vi "Source Controller.vi"() -> ()   [LabVIEW 2015]
uses:
  Type/_PIC Channel.ctl
  Type/_RT Command.ctl
  <vilib>/Utility/config.llb/Read Key (Boolean).vi
  <vilib>/Utility/config.llb/Read Key (I32).vi
  <vilib>/Utility/config.llb/Write Key (Boolean).vi
  <vilib>/Utility/config.llb/Write Key (U32).vi
  <vilib>/Utility/config.llb/NI_LVConfig.lvlib
panel:
  out "Src 2 -HV Mon":u16
  in  "Source 2 -HV":u16
  out "Src 1 -HV Mon":u16
  in  "Source 1 -HV":u16
  out "Curtain-HV Mon":u16
  in  "Curtain Cap -HV":u16
  out "Corona-HV Mon":u16
  in  "Corona -HV":u16
  out "Test":bool
  out "quit":bool
  in  "Test Channel":T1(ring)
  out "Current Cycle #":i32
  in  "# of Cycles":i32=100
  in  "Ramp Down T (mS)":u32=100
  in  "Ramp Up T (mS)":u32=100
  in  "Start Test":bool
  in  "CEM Pol":bool
  out "String":string
  in  "Pol Switch":bool
  in  "Current Channel":T2
  out "I/O Port Hd 4":u16 format="%.0x"
  out "I/O Port 4 Mon":u16
  in  "Time Const 4":u16
  out "I/O Port Hd 3":u16 format="%.0x"
  out "I/O Port 3 Mon":u16
  in  "Time Const 3":u16
  out "I/O Port Hd 2":u16 format="%.0x"
  out "I/O Port 2 Mon":u16
  in  "Time Const 2":u16
  out "I/O Port Hd 1":u16 format="%.0x"
  out "I/O Port 1 Mon":u16
  in  "Time Const 1":u16
  out "Source 2 Temp Hd":u16 format="%.0x"
  out "Source 2 HV Hd":u16 format="%.0x"
  out "Source 1 Temp Hd":u16 format="%.0x"
  out "Source 1 HV Hd":u16 format="%.0x"
  out "Curtain Cap HV Hd":u16 format="%.0x"
  out "HSID Temp Hd":u16 format="%.0x"
  out "Corona HV Hd":u16 format="%.0x"
  out "Src 2 Temp Mon":u16
  in  "Source 2 Temp":u16
  out "Src 2 +HV Mon":u16
  in  "Source 2 +HV":u16
  out "Src 1 Temp Mon":u16
  in  "Source 1 Temp":u16
  out "Src 1 +HV Mon":u16
  in  "Source 2 Pol":bool
  in  "Source 1 Pol":bool
  in  "Update All":bool
  in  "Source 1 +HV":u16
  out "Curtain+HV Mon":u16
  in  "Curtain Cap +HV":u16
  out "HSID Temp Mon":u16
  in  "HSID Temp":u16
  out "Corona+HV Mon":u16
  in  "Curtain Cap Pol":bool
  in  "Corona Pol":bool
  in  "EL":bool=TRUE
  in  "Update 1":bool
  in  "Corona +HV":u16
  in  "RP":bool=TRUE
  in  "Abort Test":bool
  # "HSID"
  # "Dual Source"
  # "HV Switch Test"
  # "Choose a Test Channel and enter the test voltages in the appropriate boxes above then press Start Test"
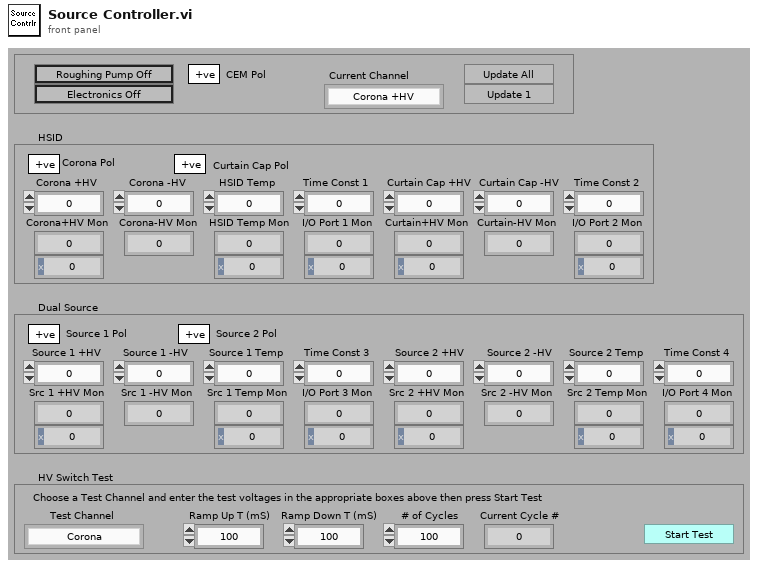
[diagram p1: front panel]
types:
  T1 = enum16{"Corona", "Curtain Cap", "Source 1", "Source 2"}
  T2 = typedef "_PIC Channel.ctl" = enum16{"Corona +HV", "Corona -HV", "HSID Temp", "Time Const 1", "Curtain Cap +HV", "Curtain Cap -HV", "Time Const 2", "Source 1 +HV", "Source 1 -HV", "Source 1 Temp", "Time Const 3", "Source 2 +HV", "Source 2 -HV", "Source 2 Temp", "Time Const 4"}
  T3 = typedef "_RT Command.ctl" = enum16{"xml Start Run", "xml Start Actual Run", "xml Stop Run", "xml Runtime Update", "xml Get Status", "xml Get Table", "xml Set Table", "xml Get Configuration", "xml System Status", "xml Set LC Input Logic", "xml Get Data", "xml Get Info", "Start", "StartActualRun", "Stop", "Runtime Update", "Get Data", "Get Info", "Get Status", "Get Param", "Get Config", "Get Table", "Read ADC", "Set Oscillator", "Update Config", "Update Table", "Set All Pol", "Set Pol and DC", "Set Max Mass", "Toggle RP", "Toggle EL", "Set PIC", "Initialize Turbo", "Send Turbo Comm", "Close Turbo", "P1", "P2", "P3", "Send Serial", "Set LC Out", "Get LC In", "Read VAC", "Test Table", "Toggle Power", "Get Startup", "Set Startup", "Get ADC Table", "Set ADC Table", "Get Brief Status", "Get Detail Status", "Auxiliary Update", "Set CC Logics", "Set CC Input Logics", "Ignore Error", "invalid"}
  T4 = typedef "NI_LVConfig.lvlib/Config Data RefNum.ctl" = refnum<k1>
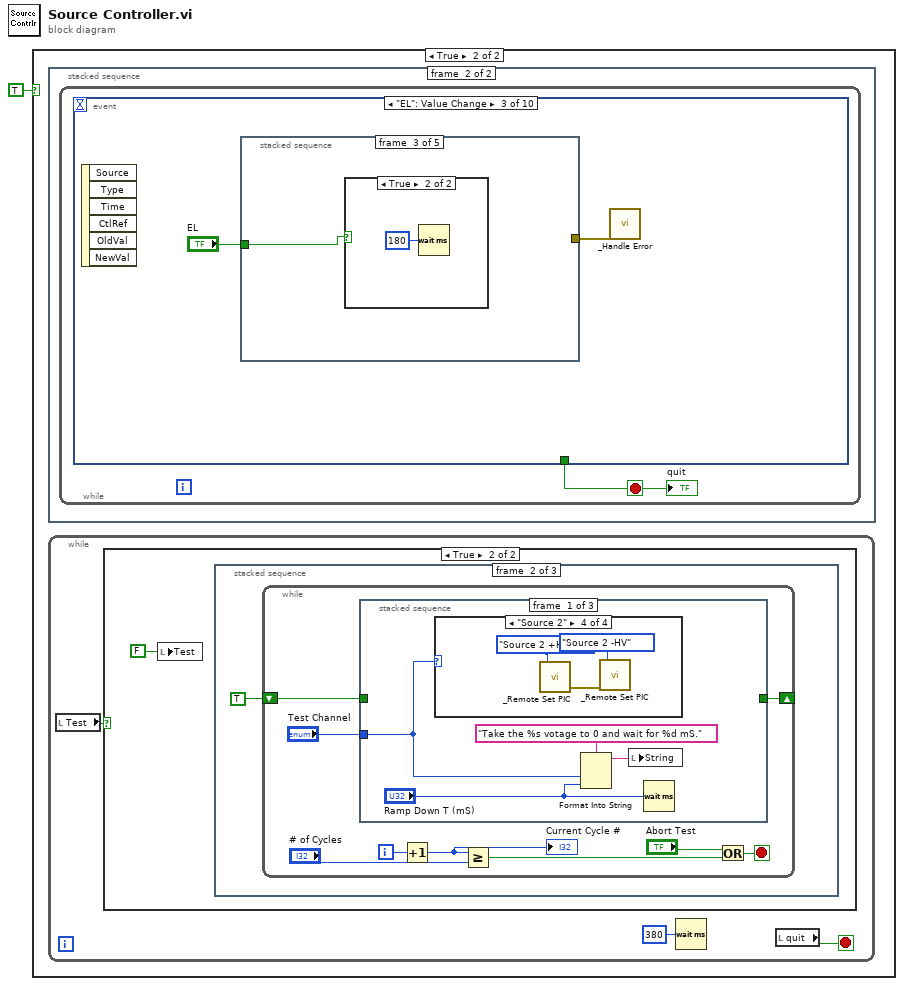
[diagram p0: block diagram]
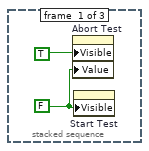
[diagram p4: hidden frame]
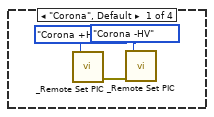
[diagram p5: hidden frame]
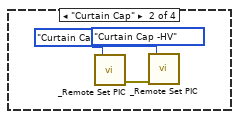
[diagram p6: hidden frame]
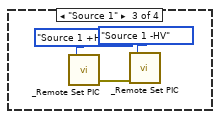
[diagram p7: hidden frame]
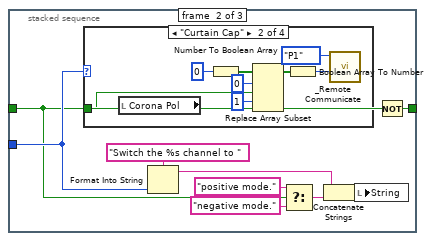
[diagram p8: hidden frame]
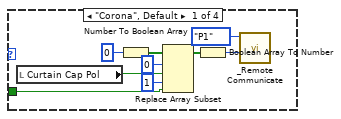
[diagram p9: hidden frame]
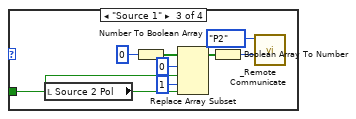
[diagram p10: hidden frame]
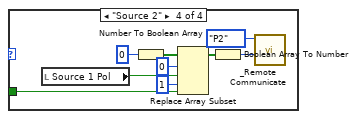
[diagram p11: hidden frame]
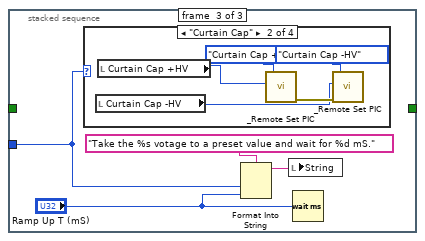
[diagram p12: hidden frame]
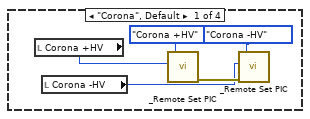
[diagram p13: hidden frame]
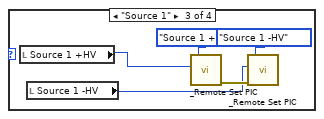
[diagram p14: hidden frame]
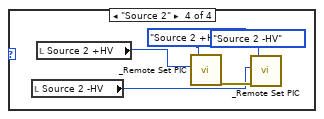
[diagram p15: hidden frame]
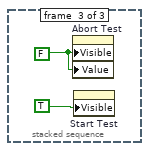
[diagram p16: hidden frame]
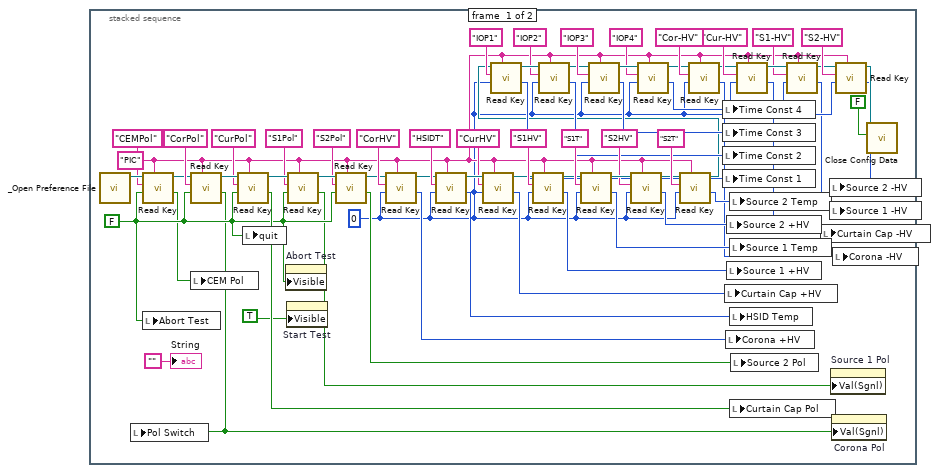
[diagram p17: hidden frame]
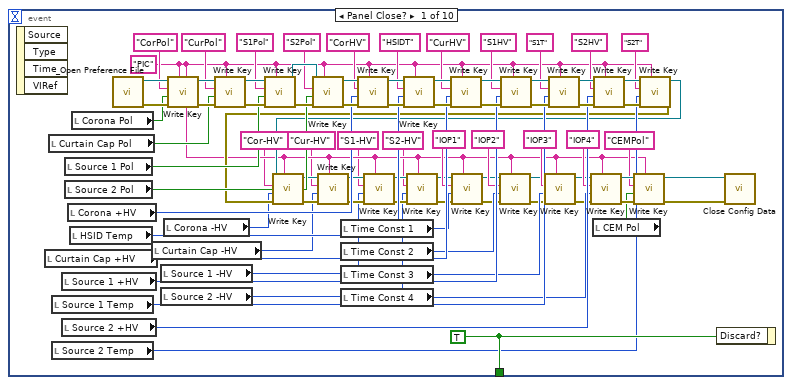
[diagram p18: hidden frame]
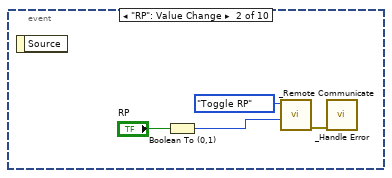
[diagram p19: hidden frame]
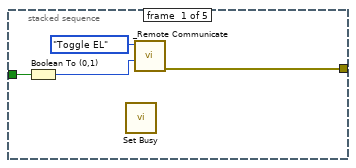
[diagram p20: hidden frame]
diagram:
  n1 = case shown="True" TRUE {
    frame False {
    }
    frame True {
      n2 = stacked-sequence {
        frame #0 {
          w123 = FALSE
          w112 = 0
          w114 = "PIC" ("section")
          n3 = call "_Open Preference File.vi"() -> ("refnum"=w128:T4)  [unwired: 3 in, 4 out]
          n4 = call-poly <vilib>:"Read Key.vi"("section"=w114, "default value"=w123, "key"="CEMPol" ("section"), "refnum"=w128) -> ("value"=w107:bool, "refnum out"=w127:T4)  [unwired: 1 in, 5 out]
          n5 = local write "Abort Test"(w123) -> ()
          n6 = call-poly <vilib>:"Read Key.vi"("section"=w114, "default value"=w123, "key"="CorPol" ("section"), "refnum"=w127) -> ("value"=w106:bool, "refnum out"=w170:T4)  [unwired: 1 in, 5 out]
          n7 = local write "Pol Switch"(w106) -> ()
          n8 = local write "CEM Pol"(w107) -> ()
          n9 = call-poly <vilib>:"Read Key.vi"("section"=w114, "default value"=w123, "key"="CurPol" ("section"), "refnum"=w170) -> ("value"=w142:bool, "refnum out"=w169:T4)  [unwired: 1 in, 5 out]
          n10 = local write "quit"(w123) -> ()
          n11 = property on="Abort Test" class="Bool (strict)"("Visible"=w123) -> ()  [unwired: 2 in, 2 out]
          n12 = property on="Start Test" class="Bool"("Visible"=TRUE) -> ()  [unwired: 2 in, 2 out]
          n13 = call-poly <vilib>:"Read Key.vi"("section"=w114, "default value"=w123, "key"="S1Pol" ("section"), "refnum"=w169) -> ("value"=w105:bool, "refnum out"=w168:T4)  [unwired: 1 in, 5 out]
          n14 = call-poly <vilib>:"Read Key.vi"("section"=w114, "default value"=w123, "key"="S2Pol" ("section"), "refnum"=w168) -> ("value"=w143:bool, "refnum out"=w162:T4)  [unwired: 1 in, 5 out]
          n15 = call-poly <vilib>:"Read Key.vi"("section"=w114, "default value"=w112, "key"="CorHV" ("section"), "refnum"=w162) -> ("value"=w144:i32, "refnum out"=w153:T4)  [unwired: 1 in, 5 out]
          n16 = call-poly <vilib>:"Read Key.vi"("section"=w114, "default value"=w112, "key"="HSIDT" ("section"), "refnum"=w153) -> ("value"=w145:i32, "refnum out"=w155:T4)  [unwired: 1 in, 5 out]
          n17 = call-poly <vilib>:"Read Key.vi"("section"=w114, "default value"=w112, "key"="CurHV" ("section"), "refnum"=w155) -> ("value"=w146:i32, "refnum out"=w156:T4)  [unwired: 1 in, 5 out]
          n18 = call-poly <vilib>:"Read Key.vi"("section"=w114, "default value"=w112, "key"="S1HV" ("section"), "refnum"=w156) -> ("value"=w147:i32, "refnum out"=w157:T4)  [unwired: 1 in, 5 out]
          n19 = call-poly <vilib>:"Read Key.vi"("section"=w114, "default value"=w112, "key"="S1T" ("section"), "refnum"=w157) -> ("value"=w148:i32, "refnum out"=w161:T4)  [unwired: 1 in, 5 out]
          n20 = call-poly <vilib>:"Read Key.vi"("section"=w114, "default value"=w112, "key"="S2HV" ("section"), "refnum"=w161) -> ("value"=w149:i32, "refnum out"=w151:T4)  [unwired: 1 in, 5 out]
          n21 = call-poly <vilib>:"Read Key.vi"("section"=w114, "default value"=w112, "key"="S2T" ("section"), "refnum"=w151) -> ("value"=w150:i32, "refnum out"=w130:T4)  [unwired: 1 in, 5 out]
          n22 = call-poly <vilib>:"Read Key.vi"("section"=w114, "default value"=w112, "key"="IOP1" ("section"), "refnum"=w130) -> ("value"=w131:i32, "refnum out"=w139:T4)  [unwired: 1 in, 5 out]
          n23 = call-poly <vilib>:"Read Key.vi"("section"=w114, "default value"=w112, "key"="IOP2" ("section"), "refnum"=w139) -> ("value"=w132:i32, "refnum out"=w135:T4)  [unwired: 1 in, 5 out]
          n24 = call-poly <vilib>:"Read Key.vi"("section"=w114, "default value"=w112, "key"="IOP3" ("section"), "refnum"=w135) -> ("value"=w133:i32, "refnum out"=w141:T4)  [unwired: 1 in, 5 out]
          n25 = call-poly <vilib>:"Read Key.vi"("section"=w114, "default value"=w112, "key"="IOP4" ("section"), "refnum"=w141) -> ("value"=w125:i32, "refnum out"=w115:T4)  [unwired: 1 in, 5 out]
          n26 = call-poly <vilib>:"Read Key.vi"("section"=w114, "default value"=w112, "key"="Cor-HV" ("section"), "refnum"=w115) -> ("value"=w108:i32, "refnum out"=w118:T4)  [unwired: 1 in, 5 out]
          n27 = local write "Time Const 4"(w125) -> ()
          n28 = local write "Time Const 3"(w133) -> ()
          n29 = local write "Time Const 2"(w132) -> ()
          n30 = local write "Time Const 1"(w131) -> ()
          n31 = local write "Curtain Cap +HV"(w146) -> ()
          n32 = local write "Corona +HV"(w144) -> ()
          n33 = local write "Source 2 +HV"(w149) -> ()
          n34 = local write "Source 1 +HV"(w147) -> ()
          n35 = local write "Source 2 Temp"(w150) -> ()
          n36 = local write "Source 1 Temp"(w148) -> ()
          n37 = local write "HSID Temp"(w145) -> ()
          n38 = local write "Curtain Cap Pol"(w142) -> ()
          n39 = local write "Source 2 Pol"(w143) -> ()
          n40 = call-poly <vilib>:"Read Key.vi"("section"=w114, "default value"=w112, "key"="Cur-HV" ("section"), "refnum"=w118) -> ("value"=w109:i32, "refnum out"=w122:T4)  [unwired: 1 in, 5 out]
          n41 = call-poly <vilib>:"Read Key.vi"("section"=w114, "default value"=w112, "key"="S1-HV" ("section"), "refnum"=w122) -> ("value"=w110:i32, "refnum out"=w116:T4)  [unwired: 1 in, 5 out]
          n42 = local write "Curtain Cap -HV"(w109) -> ()
          n43 = local write "Source 1 -HV"(w110) -> ()
          n44 = property on="Source 1 Pol" class="Bool (strict)"("Val(Sgnl)"=w105) -> ()  [unwired: 2 in, 2 out]
          n45 = property on="Corona Pol" class="Bool (strict)"("Val(Sgnl)"=w106) -> ()  [unwired: 2 in, 2 out]
          n46 = local write "Corona -HV"(w108) -> ()
          n47 = call-poly <vilib>:"Read Key.vi"("section"=w114, "default value"=w112, "key"="S2-HV" ("section"), "refnum"=w116) -> ("value"=w111:i32, "refnum out"=w113:T4)  [unwired: 1 in, 5 out]
          n48 = local write "Source 2 -HV"(w111) -> ()
          n49 = call <vilib>:"Close Config Data.vi"("write file if changed (T)"=FALSE ("write configuration file? (T)"), "refnum"=w113) -> ()  [unwired: 1 in, 9 out]
          "String" <- ""
        }
        frame #1 {
          n50 = while {
            stop <- w172 stop-if-true
            n51 = event shown="[2] \"EL\": Value Change" {
              selector: _ -> [_ _ _ _ _ _ _ _ _ _]
              dyn-events: _ -> [_ _ _ _ _ _ _ _ _ _]
              timeout: _ -> [_ _ _ _ _ _ _ _ _ _]
              tunnel: [w256 _ _ _ _ _ _ _ _ _] -> w172
              event Panel Close? {
                w181 = "PIC" ("section")
                w256 = TRUE
                n52 = event-data() -> ()  [unwired: 5 out]
                n53 = local read "Curtain Cap +HV"() -> (w216:u16)
                n54 = local read "Curtain Cap Pol"() -> (w221:bool)
                n55 = local read "Source 1 Temp"() -> (w214:u16)
                n56 = local read "Source 2 Temp"() -> (w212:u16)
                n57 = local read "Source 1 +HV"() -> (w215:u16)
                n58 = local read "Source 2 +HV"() -> (w213:u16)
                n59 = local read "Source 1 Pol"() -> (w220:bool)
                n60 = local read "Source 2 Pol"() -> (w219:bool)
                n61 = local read "Corona +HV"() -> (w218:u16)
                n62 = local read "HSID Temp"() -> (w217:u16)
                n63 = local read "Corona Pol"() -> (w222:bool)
                n64 = call "_Open Preference File.vi"() -> ("error"=w252:errorcluster, "refnum"=w251:T4)  [unwired: 3 in, 3 out]
                n65 = local read "Curtain Cap -HV"() -> (w175:u16)
                n66 = local read "Source 1 -HV"() -> (w174:u16)
                n67 = local read "Source 2 -HV"() -> (w173:u16)
                n68 = local read "Corona -HV"() -> (w176:u16)
                n69 = call-poly <vilib>:"Write Key.vi"("section"=w181, "error in (no error)"=w252, "value"=w222, "key"="CorPol" ("section"), "refnum"=w251) -> ("error out"=w253:errorcluster, "refnum out"=w250:T4)  [unwired: 5 out]
                n70 = call-poly <vilib>:"Write Key.vi"("section"=w181, "error in (no error)"=w253, "value"=w221, "key"="CurPol" ("section"), "refnum"=w250) -> ("error out"=w254:errorcluster, "refnum out"=w249:T4)  [unwired: 5 out]
                n71 = call-poly <vilib>:"Write Key.vi"("section"=w181, "error in (no error)"=w254, "value"=w220, "key"="S1Pol" ("section"), "refnum"=w249) -> ("error out"=w255:errorcluster, "refnum out"=w248:T4)  [unwired: 5 out]
                n72 = call-poly <vilib>:"Write Key.vi"("section"=w181, "error in (no error)"=w255, "value"=w219, "key"="S2Pol" ("section"), "refnum"=w248) -> ("error out"=w246:errorcluster, "refnum out"=w247:T4)  [unwired: 5 out]
                n73 = local read "Time Const 1"() -> (w204:u16)
                n74 = local read "Time Const 2"() -> (w203:u16)
                n75 = local read "Time Const 3"() -> (w202:u16)
                n76 = local read "Time Const 4"() -> (w201:u16)
                n77 = call-poly <vilib>:"Write Key.vi"("section"=w181, "error in (no error)"=w246, "value"=w218, "key"="CorHV" ("section"), "refnum"=w247) -> ("error out"=w237:errorcluster, "refnum out"=w236:T4)  [unwired: 5 out]
                n78 = call-poly <vilib>:"Write Key.vi"("section"=w181, "error in (no error)"=w237, "value"=w217, "key"="HSIDT" ("section"), "refnum"=w236) -> ("error out"=w240:errorcluster, "refnum out"=w241:T4)  [unwired: 5 out]
                n79 = call-poly <vilib>:"Write Key.vi"("section"=w181, "error in (no error)"=w240, "value"=w216, "key"="CurHV" ("section"), "refnum"=w241) -> ("error out"=w239:errorcluster, "refnum out"=w242:T4)  [unwired: 5 out]
                n80 = call-poly <vilib>:"Write Key.vi"("section"=w181, "error in (no error)"=w239, "value"=w215, "key"="S1HV" ("section"), "refnum"=w242) -> ("error out"=w238:errorcluster, "refnum out"=w243:T4)  [unwired: 5 out]
                n81 = call-poly <vilib>:"Write Key.vi"("section"=w181, "error in (no error)"=w238, "value"=w214, "key"="S1T" ("section"), "refnum"=w243) -> ("error out"=w245:errorcluster, "refnum out"=w244:T4)  [unwired: 5 out]
                n82 = local read "CEM Pol"() -> (w194:bool)
                n83 = call-poly <vilib>:"Write Key.vi"("section"=w181, "error in (no error)"=w245, "value"=w213, "key"="S2HV" ("section"), "refnum"=w244) -> ("error out"=w235:errorcluster, "refnum out"=w234:T4)  [unwired: 5 out]
                n84 = call-poly <vilib>:"Write Key.vi"("section"=w181, "error in (no error)"=w235, "value"=w212, "key"="S2T" ("section"), "refnum"=w234) -> ("error out"=w184:errorcluster, "refnum out"=w183:T4)  [unwired: 5 out]
                n85 = call-poly <vilib>:"Write Key.vi"("section"=w181, "error in (no error)"=w184, "value"=w176, "key"="Cor-HV" ("section"), "refnum"=w183) -> ("error out"=w191:errorcluster, "refnum out"=w190:T4)  [unwired: 5 out]
                n86 = call-poly <vilib>:"Write Key.vi"("section"=w181, "error in (no error)"=w191, "value"=w175, "key"="Cur-HV" ("section"), "refnum"=w190) -> ("error out"=w186:errorcluster, "refnum out"=w187:T4)  [unwired: 5 out]
                n87 = call-poly <vilib>:"Write Key.vi"("section"=w181, "error in (no error)"=w186, "value"=w174, "key"="S1-HV" ("section"), "refnum"=w187) -> ("error out"=w189:errorcluster, "refnum out"=w188:T4)  [unwired: 5 out]
                n88 = call-poly <vilib>:"Write Key.vi"("section"=w181, "error in (no error)"=w189, "value"=w173, "key"="S2-HV" ("section"), "refnum"=w188) -> ("error out"=w185:errorcluster, "refnum out"=w182:T4)  [unwired: 5 out]
                n89 = call-poly <vilib>:"Write Key.vi"("section"=w181, "error in (no error)"=w185, "value"=w204, "key"="IOP1" ("section"), "refnum"=w182) -> ("error out"=w200:errorcluster, "refnum out"=w206:T4)  [unwired: 5 out]
                n90 = call-poly <vilib>:"Write Key.vi"("section"=w181, "error in (no error)"=w200, "value"=w203, "key"="IOP2" ("section"), "refnum"=w206) -> ("error out"=w199:errorcluster, "refnum out"=w205:T4)  [unwired: 5 out]
                n91 = call-poly <vilib>:"Write Key.vi"("section"=w181, "error in (no error)"=w199, "value"=w202, "key"="IOP3" ("section"), "refnum"=w205) -> ("error out"=w198:errorcluster, "refnum out"=w207:T4)  [unwired: 5 out]
                n92 = call-poly <vilib>:"Write Key.vi"("section"=w181, "error in (no error)"=w198, "value"=w201, "key"="IOP4" ("section"), "refnum"=w207) -> ("error out"=w196:errorcluster, "refnum out"=w197:T4)  [unwired: 5 out]
                n93 = call-poly <vilib>:"Write Key.vi"("section"=w181, "error in (no error)"=w196, "value"=w194, "key"="CEMPol" ("section"), "refnum"=w197) -> ("error out"=w192:errorcluster, "refnum out"=w193:T4)  [unwired: 5 out]
                n94 = event-data("Discard?"=w256) -> ()  [unwired: 1 in, 1 out]
                n95 = call <vilib>:"Close Config Data.vi"("error in (no error)"=w192, "refnum"=w193) -> ()  [unwired: 1 in, 9 out]
              }
              event "RP": Value Change {
                n96 = event-data() -> ()  [unwired: 2 out]
                n97 = Boolean To (0,1)(Boolean="RP") -> (0, 1=w257:i16)
                n98 = call "_Remote Communicate.vi"("DC Param"=w257, "Command"=_RT_Command."Toggle RP") -> ("error out"=w259:errorcluster)  [unwired: 4 in, 3 out]
                n99 = call "_Handle Error.vi"("error in (no error)"=w259) -> ()  [unwired: 2 in, 5 out]
              }
              event "EL": Value Change {
                n100 = event-data() -> ()  [unwired: 7 out]
                n101 = stacked-sequence {
                  tunnel: "EL" -> [w265 w267 w270 w272 _]
                  tunnel: [w263 _ _ _ _] -> w261
                  frame #0 {
                    n102 = Boolean To (0,1)(Boolean=w265) -> (0, 1=w264:i16)
                    n103 = call <vilib>:"Set Busy.vi"() -> ()  [unwired: 4 in, 8 out]
                    n104 = call "_Remote Communicate.vi"("DC Param"=w264, "Command"=_RT_Command."Toggle EL") -> ("error out"=w263:errorcluster)  [unwired: 4 in, 3 out]
                  }
                  frame #1 {
                    n105 = case shown="True" w267 {
                      frame False {
                      }
                      frame True {
                        n106 = call "_Remote Park Lens.vi"("All Ch (F)"=TRUE) -> ("error out"=w268:errorcluster)  [unwired: 1 in, 5 out]
                        n107 = call "_Remote Program Oscil.vi"("error in (no error)"=w268) -> ()  [unwired: 1 out]
                      }
                    }
                  }
                  frame #2 {
                    n108 = case shown="True" w270 {
                      frame False {
                      }
                      frame True {
                        n109 = Wait (ms)(milliseconds to wait=u32 180) -> ()  [unwired: 1 out]
                      }
                    }
                  }
                  frame #3 {
                    n110 = case shown="True" w272 {
                      frame False {
                      }
                      frame True {
                        n111 = call "_Remote Park Lens.vi"("All Ch (F)"=TRUE) -> ("error out"=w273:errorcluster)  [unwired: 1 in, 5 out]
                        n112 = call "_Remote Program Oscil.vi"("error in (no error)"=w273) -> ()  [unwired: 1 out]
                      }
                    }
                  }
                  frame #4 {
                    n113 = call <vilib>:"Unset Busy.vi"() -> ()  [unwired: 2 in, 10 out]
                  }
                }
                n114 = call "_Handle Error.vi"("error in (no error)"=w261) -> ()  [unwired: 2 in, 5 out]
              }
              event "Update 1": Value Change {
                n115 = event-data() -> ()  [unwired: 7 out]
                n116 = stacked-sequence {
                  tunnel: [_ w280 _] -> w275
                  frame #0 {
                    n117 = call <vilib>:"Set Busy.vi"() -> ()  [unwired: 4 in, 8 out]
                  }
                  frame #1 {
                    n118 = case shown="\"Corona +HV\", Default" "Current Channel" {
                      tunnel: [w311 w312 w313 w314 w315 w316 w317 w318 w319 w320 w321 w322 w323 w324 w325] -> w276
                      frame "Corona +HV", Default {
                        n119 = local read "Corona +HV"() -> (w311:u16)
                      }
                      frame "Corona -HV" {
                        n120 = local read "Corona -HV"() -> (w312:u16)
                      }
                      frame "HSID Temp" {
                        n121 = local read "HSID Temp"() -> (w313:u16)
                      }
                      frame "Time Const 1" {
                        n122 = local read "Time Const 1"() -> (w314:u16)
                      }
                      frame "Curtain Cap +HV" {
                        n123 = local read "Curtain Cap +HV"() -> (w315:u16)
                      }
                      frame "Curtain Cap -HV" {
                        n124 = local read "Curtain Cap -HV"() -> (w316:u16)
                      }
                      frame "Time Const 2" {
                        n125 = local read "Time Const 2"() -> (w317:u16)
                      }
                      frame "Source 1 +HV" {
                        n126 = local read "Source 1 +HV"() -> (w318:u16)
                      }
                      frame "Source 1 -HV" {
                        n127 = local read "Source 1 -HV"() -> (w319:u16)
                      }
                      frame "Source 1 Temp" {
                        n128 = local read "Source 1 Temp"() -> (w320:u16)
                      }
                      frame "Time Const 3" {
                        n129 = local read "Time Const 3"() -> (w321:u16)
                      }
                      frame "Source 2 +HV" {
                        n130 = local read "Source 2 +HV"() -> (w322:u16)
                      }
                      frame "Source 2 -HV" {
                        n131 = local read "Source 2 -HV"() -> (w323:u16)
                      }
                      frame "Source 2 Temp" {
                        n132 = local read "Source 2 Temp"() -> (w324:u16)
                      }
                      frame "Time Const 4" {
                        n133 = local read "Time Const 4"() -> (w325:u16)
                      }
                    }
                    n134 = call "_Remote Set PIC.vi"("Set Value"=w276, "PIC Channel"="Current Channel") -> ("error out"=w280:errorcluster, "Received Value"=w277:u16, "Received Header"=w278:u16)  [unwired: 1 in, 2 out]
                    n135 = case shown="\"Source 2 Temp\"" "Current Channel" {
                      tunnel: w278 -> [w282 w284 w286 w288 w290 w292 w294 w296 w298 w300 w302 w304 w306 w308 w310]
                      tunnel: w277 -> [w281 w283 w285 w287 w289 w291 w293 w295 w297 w299 w301 w303 w305 w307 w309]
                      frame "Corona +HV", Default {
                        n136 = local write "Corona HV Hd"(w282) -> ()
                        n137 = local write "Corona+HV Mon"(w281) -> ()
                      }
                      frame "Corona -HV" {
                        n138 = local write "Corona HV Hd"(w284) -> ()
                        n139 = local write "Corona-HV Mon"(w283) -> ()
                      }
                      frame "HSID Temp" {
                        n140 = local write "HSID Temp Mon"(w285) -> ()
                        n141 = local write "HSID Temp Hd"(w286) -> ()
                      }
                      frame "Time Const 1" {
                        n142 = local write "I/O Port 1 Mon"(w287) -> ()
                        n143 = local write "I/O Port Hd 1"(w288) -> ()
                      }
                      frame "Curtain Cap +HV" {
                        n144 = local write "Curtain Cap HV Hd"(w290) -> ()
                        n145 = local write "Curtain+HV Mon"(w289) -> ()
                      }
                      frame "Curtain Cap -HV" {
                        n146 = local write "Curtain Cap HV Hd"(w292) -> ()
                        n147 = local write "Curtain-HV Mon"(w291) -> ()
                      }
                      frame "Time Const 2" {
                        n148 = local write "I/O Port 2 Mon"(w293) -> ()
                        n149 = local write "I/O Port Hd 2"(w294) -> ()
                      }
                      frame "Source 1 +HV" {
                        n150 = local write "Source 1 HV Hd"(w296) -> ()
                        n151 = local write "Src 1 +HV Mon"(w295) -> ()
                      }
                      frame "Source 1 -HV" {
                        n152 = local write "Source 1 HV Hd"(w298) -> ()
                        n153 = local write "Src 1 -HV Mon"(w297) -> ()
                      }
                      frame "Source 1 Temp" {
                        n154 = local write "Source 1 Temp Hd"(w300) -> ()
                        n155 = local write "Src 1 Temp Mon"(w299) -> ()
                      }
                      frame "Time Const 3" {
                        n156 = local write "I/O Port 3 Mon"(w301) -> ()
                        n157 = local write "I/O Port Hd 3"(w302) -> ()
                      }
                      frame "Source 2 +HV" {
                        n158 = local write "Source 2 HV Hd"(w304) -> ()
                        n159 = local write "Src 2 +HV Mon"(w303) -> ()
                      }
                      frame "Source 2 -HV" {
                        n160 = local write "Source 2 HV Hd"(w306) -> ()
                        n161 = local write "Src 2 -HV Mon"(w305) -> ()
                      }
                      frame "Source 2 Temp" {
                        n162 = local write "Source 2 Temp Hd"(w308) -> ()
                        n163 = local write "Src 2 Temp Mon"(w307) -> ()
                      }
                      frame "Time Const 4" {
                        n164 = local write "I/O Port 4 Mon"(w309) -> ()
                        n165 = local write "I/O Port Hd 4"(w310) -> ()
                      }
                    }
                  }
                  frame #2 {
                    n166 = call <vilib>:"Unset Busy.vi"() -> ()  [unwired: 2 in, 10 out]
                  }
                }
                n167 = call "_Handle Error.vi"("error in (no error)"=w275) -> ()  [unwired: 2 in, 5 out]
              }
              event "Update All": Value Change {
                n168 = event-data() -> ()  [unwired: 7 out]
                n169 = stacked-sequence {
                  frame #0 {
                    n170 = call <vilib>:"Set Busy.vi"() -> ()  [unwired: 4 in, 8 out]
                  }
                  frame #1 {
                    n171 = call "_Remote Set PIC.vi"("Set Value"="Corona +HV", "PIC Channel"=_PIC_Channel."Corona +HV") -> ("Received Value"=→"Corona+HV Mon":u16, "Received Header"=→"Corona HV Hd":u16)  [unwired: 1 in, 3 out]
                  }
                  frame #2 {
                    n172 = call "_Remote Set PIC.vi"("Set Value"="Corona -HV", "PIC Channel"=_PIC_Channel."Corona -HV") -> ("Received Value"=→"Corona-HV Mon":u16, "Received Header"=w330:u16)  [unwired: 1 in, 3 out]
                    n173 = local write "Corona HV Hd"(w330) -> ()
                  }
                  frame #3 {
                    n174 = call "_Remote Set PIC.vi"("Set Value"="HSID Temp", "PIC Channel"=_PIC_Channel."HSID Temp") -> ("Received Value"=→"HSID Temp Mon":u16, "Received Header"=→"HSID Temp Hd":u16)  [unwired: 1 in, 3 out]
                  }
                  frame #4 {
                    n175 = call "_Remote Set PIC.vi"("Set Value"="Time Const 1", "PIC Channel"=_PIC_Channel."Time Const 1") -> ("Received Value"=→"I/O Port 1 Mon":u16, "Received Header"=→"I/O Port Hd 1":u16)  [unwired: 1 in, 3 out]
                  }
                  frame #5 {
                    n176 = call "_Remote Set PIC.vi"("Set Value"="Curtain Cap +HV", "PIC Channel"=_PIC_Channel."Curtain Cap +HV") -> ("Received Value"=→"Curtain+HV Mon":u16, "Received Header"=→"Curtain Cap HV Hd":u16)  [unwired: 1 in, 3 out]
                  }
                  frame #6 {
                    n177 = call "_Remote Set PIC.vi"("Set Value"="Curtain Cap -HV", "PIC Channel"=_PIC_Channel."Curtain Cap -HV") -> ("Received Value"=→"Curtain-HV Mon":u16, "Received Header"=w347:u16)  [unwired: 1 in, 3 out]
                    n178 = local write "Curtain Cap HV Hd"(w347) -> ()
                  }
                  frame #7 {
                    n179 = call "_Remote Set PIC.vi"("Set Value"="Time Const 2", "PIC Channel"=_PIC_Channel."Time Const 2") -> ("Received Value"=→"I/O Port 2 Mon":u16, "Received Header"=→"I/O Port Hd 2":u16)  [unwired: 1 in, 3 out]
                  }
                  frame #8 {
                    n180 = call "_Remote Set PIC.vi"("Set Value"="Source 1 +HV", "PIC Channel"=_PIC_Channel."Source 1 +HV") -> ("Received Value"=→"Src 1 +HV Mon":u16, "Received Header"=→"Source 1 HV Hd":u16)  [unwired: 1 in, 3 out]
                  }
                  frame #9 {
                    n181 = call "_Remote Set PIC.vi"("Set Value"="Source 1 -HV", "PIC Channel"=_PIC_Channel."Source 1 -HV") -> ("Received Value"=→"Src 1 -HV Mon":u16, "Received Header"=w359:u16)  [unwired: 1 in, 3 out]
                    n182 = local write "Source 1 HV Hd"(w359) -> ()
                  }
                  frame #10 {
                    n183 = call "_Remote Set PIC.vi"("Set Value"="Source 1 Temp", "PIC Channel"=_PIC_Channel."Source 1 Temp") -> ("Received Value"=→"Src 1 Temp Mon":u16, "Received Header"=→"Source 1 Temp Hd":u16)  [unwired: 1 in, 3 out]
                  }
                  frame #11 {
                    n184 = call "_Remote Set PIC.vi"("Set Value"="Time Const 3", "PIC Channel"=_PIC_Channel."Time Const 3") -> ("Received Value"=→"I/O Port 3 Mon":u16, "Received Header"=→"I/O Port Hd 3":u16)  [unwired: 1 in, 3 out]
                  }
                  frame #12 {
                    n185 = call "_Remote Set PIC.vi"("Set Value"="Source 2 +HV", "PIC Channel"=_PIC_Channel."Source 2 +HV") -> ("Received Value"=→"Src 2 +HV Mon":u16, "Received Header"=→"Source 2 HV Hd":u16)  [unwired: 1 in, 3 out]
                  }
                  frame #13 {
                    n186 = call "_Remote Set PIC.vi"("Set Value"="Source 2 -HV", "PIC Channel"=_PIC_Channel."Source 2 -HV") -> ("Received Value"=→"Src 2 -HV Mon":u16, "Received Header"=w375:u16)  [unwired: 1 in, 3 out]
                    n187 = local write "Source 1 HV Hd"(w375) -> ()
                  }
                  frame #14 {
                    n188 = call "_Remote Set PIC.vi"("Set Value"="Source 2 Temp", "PIC Channel"=_PIC_Channel."Source 2 Temp") -> ("Received Value"=→"Src 2 Temp Mon":u16, "Received Header"=→"Source 2 Temp Hd":u16)  [unwired: 1 in, 3 out]
                  }
                  frame #15 {
                    n189 = call "_Remote Set PIC.vi"("Set Value"="Time Const 4", "PIC Channel"=_PIC_Channel."Time Const 4") -> ("Received Value"=→"I/O Port 4 Mon":u16, "Received Header"=→"I/O Port Hd 4":u16)  [unwired: 1 in, 3 out]
                  }
                  frame #16 {
                    n190 = call <vilib>:"Unset Busy.vi"() -> ()  [unwired: 2 in, 10 out]
                  }
                }
              }
              event "Pol Switch": Value Change {
                # "Obsolete"
                n191 = event-data() -> ()  [unwired: 7 out]
                n192 = stacked-sequence {
                  tunnel: "Pol Switch" -> [w387 _ _ w401 _ _]
                  frame #0 {
                    n193 = call <vilib>:"Set Busy.vi"() -> ()  [unwired: 4 in, 8 out]
                    n194 = local write "Curtain Cap Pol"(w387) -> ()
                    n195 = local write "Source 1 Pol"(w387) -> ()
                    n196 = local write "Corona Pol"(w387) -> ()
                    n197 = local write "Source 2 Pol"(w387) -> ()
                    n198 = local write "String"("Setting voltage to 0" ("String")) -> ()
                  }
                  frame #1 {
                    w389 = u16 0 ("Set Value")
                    n199 = call "_Remote Set PIC.vi"("Set Value"=w389, "PIC Channel"=_PIC_Channel."Corona +HV") -> ("error out"=w392:errorcluster)  [unwired: 1 in, 4 out]
                    n200 = call "_Remote Set PIC.vi"("error in (no error)"=w392, "Set Value"=w389, "PIC Channel"=_PIC_Channel."HSID Temp") -> ("error out"=w393:errorcluster)  [unwired: 4 out]
                    n201 = call "_Remote Set PIC.vi"("error in (no error)"=w393, "Set Value"=w389, "PIC Channel"=_PIC_Channel."Curtain Cap -HV") -> ("error out"=w394:errorcluster)  [unwired: 4 out]
                    n202 = call "_Remote Set PIC.vi"("error in (no error)"=w394, "Set Value"=w389, "PIC Channel"=_PIC_Channel."Source 1 -HV") -> ()  [unwired: 5 out]
                  }
                  frame #2 {
                    n203 = Wait (ms)(milliseconds to wait=u32 20000) -> ()  [unwired: 1 out]
                    n204 = local write "String"("Wait for 20 Sec" ("String")) -> ()
                  }
                  frame #3 {
                    n205 = Boolean To (0,1)(Boolean=w401) -> (0, 1=w400:i16)
                    n206 = local write "String"("Switching polarity" ("String")) -> ()
                    n207 = call "_Remote Communicate.vi"("DC Param"=w400, "Command"=_RT_Command."Set All Pol") -> ()  [unwired: 4 in, 4 out]
                  }
                  frame #4 {
                    n208 = local read "Curtain Cap +HV"() -> (w405:u16)
                    n209 = local read "Source 1 +HV"() -> (w404:u16)
                    n210 = local read "Source 2 +HV"() -> (w403:u16)
                    n211 = local read "Corona +HV"() -> (w406:u16)
                    n212 = call "_Remote Set PIC.vi"("Set Value"=w406, "PIC Channel"=_PIC_Channel."Corona +HV") -> ("error out"=w409:errorcluster)  [unwired: 1 in, 4 out]
                    n213 = call "_Remote Set PIC.vi"("error in (no error)"=w409, "Set Value"=w405, "PIC Channel"=_PIC_Channel."HSID Temp") -> ("error out"=w410:errorcluster)  [unwired: 4 out]
                    n214 = call "_Remote Set PIC.vi"("error in (no error)"=w410, "Set Value"=w404, "PIC Channel"=_PIC_Channel."Curtain Cap -HV") -> ("error out"=w411:errorcluster)  [unwired: 4 out]
                    n215 = call "_Remote Set PIC.vi"("error in (no error)"=w411, "Set Value"=w403, "PIC Channel"=_PIC_Channel."Source 1 -HV") -> ()  [unwired: 5 out]
                  }
                  frame #5 {
                    n216 = local write "String"("") -> ()
                    n217 = call <vilib>:"Unset Busy.vi"() -> ()  [unwired: 2 in, 10 out]
                  }
                }
              }
              event "Corona Pol", "Curtain Cap Pol": Value Change {
                n218 = event-data() -> ()  [unwired: 7 out]
                n219 = Number To Boolean Array(number=u16 0) -> (Boolean array=w422:bool[])
                n220 = Replace Array Subset(array=w422, new element #1="Curtain Cap Pol", index #1=0 ("index"), new element #2="Corona Pol", index #2=1 ("index")) -> (w419:bool[])
                n221 = Boolean Array To Number(Boolean array=w419) -> (number=w417:u16)
                n222 = call "_Remote Communicate.vi"("DC Param"=w417, "Command"=_RT_Command."P1") -> ()  [unwired: 4 in, 4 out]
              }
              event "Source 1 Pol", "Source 2 Pol": Value Change {
                n223 = event-data() -> ()  [unwired: 7 out]
                n224 = Number To Boolean Array(number=u16 0) -> (Boolean array=w431:bool[])
                n225 = Replace Array Subset(array=w431, new element #1="Source 1 Pol", index #1=0 ("index"), new element #2="Source 2 Pol", index #2=1 ("index")) -> (w428:bool[])
                n226 = Boolean Array To Number(Boolean array=w428) -> (number=w426:u16)
                n227 = call "_Remote Communicate.vi"("DC Param"=w426, "Command"=_RT_Command."P2") -> ()  [unwired: 4 in, 4 out]
              }
              event "CEM Pol": Value Change {
                n228 = event-data() -> ()  [unwired: 7 out]
                n229 = Number To Boolean Array(number=u16 0) -> (Boolean array=w439:bool[])
                n230 = Replace Array Subset(array=w439, new element #1="CEM Pol", index #1=0 ("index"), new element #2="CEM Pol", index #2=1 ("index")) -> (w436:bool[])
                n231 = Boolean Array To Number(Boolean array=w436) -> (number=w434:u16)
                n232 = call "_Remote Communicate.vi"("DC Param"=w434, "Command"=_RT_Command."P3") -> ()  [unwired: 4 in, 4 out]
              }
              event "Start Test": Value Change {
                n233 = event-data() -> ()  [unwired: 2 out]
                "Test" <- "Start Test"
              }
            }
            "quit" <- w172
          }
        }
      }
      n234 = while {
        stop <- w4 stop-if-true
        n235 = local read "Test"() -> (w2:bool)
        n236 = case shown="True" w2 {
          frame False {
          }
          frame True {
            n237 = local write "Test"(FALSE ("Test")) -> ()
            n238 = stacked-sequence {
              frame #0 {
                w6 = FALSE ("Visible")
                n239 = property on="Abort Test" class="Bool (strict)"("Visible"=TRUE, "Value"=w6) -> ()  [unwired: 2 in, 2 out]
                n240 = property on="Start Test" class="Bool"("Visible"=w6) -> ()  [unwired: 2 in, 2 out]
              }
              frame #1 {
                n241 = while {
                  shift-right: [w11] -> _
                  shift-left: TRUE -> [w12]
                  i -> [w17]
                  stop <- w16 stop-if-true
                  n242 = stacked-sequence {
                    tunnel: "Test Channel" -> [w19 w41 w80]
                    tunnel: w12 -> [_ w34 _]
                    tunnel: [_ w38 _] -> w11
                    frame #0 {
                      n243 = case shown="\"Source 2\"" w19 {
                        frame "Corona", Default {
                          n244 = call "_Remote Set PIC.vi"("PIC Channel"=_PIC_Channel."Corona +HV") -> ("error out"=w22:errorcluster)  [unwired: 2 in, 4 out]
                          n245 = call "_Remote Set PIC.vi"("error in (no error)"=w22, "PIC Channel"=_PIC_Channel."Corona -HV") -> ()  [unwired: 1 in, 5 out]
                        }
                        frame "Curtain Cap" {
                          n246 = call "_Remote Set PIC.vi"("PIC Channel"=_PIC_Channel."Curtain Cap +HV") -> ("error out"=w25:errorcluster)  [unwired: 2 in, 4 out]
                          n247 = call "_Remote Set PIC.vi"("error in (no error)"=w25, "PIC Channel"=_PIC_Channel."Curtain Cap -HV") -> ()  [unwired: 1 in, 5 out]
                        }
                        frame "Source 1" {
                          n248 = call "_Remote Set PIC.vi"("PIC Channel"=_PIC_Channel."Source 1 +HV") -> ("error out"=w28:errorcluster)  [unwired: 2 in, 4 out]
                          n249 = call "_Remote Set PIC.vi"("error in (no error)"=w28, "PIC Channel"=_PIC_Channel."Source 1 -HV") -> ()  [unwired: 1 in, 5 out]
                        }
                        frame "Source 2" {
                          n250 = call "_Remote Set PIC.vi"("PIC Channel"=_PIC_Channel."Source 2 +HV") -> ("error out"=w31:errorcluster)  [unwired: 2 in, 4 out]
                          n251 = call "_Remote Set PIC.vi"("error in (no error)"=w31, "PIC Channel"=_PIC_Channel."Source 2 -HV") -> ()  [unwired: 1 in, 5 out]
                        }
                      }
                      n252 = Format Into String(format string="Take the %s votage to 0 and wait for %d mS.", w19, "Ramp Down T (mS)") -> (resulting string=w20:string)  [unwired: 2 in, 1 out]
                      n253 = local write "String"(w20) -> ()
                      n254 = Wait (ms)(milliseconds to wait="Ramp Down T (mS)") -> ()  [unwired: 1 out]
                    }
                    frame #1 {
                      n255 = case shown="\"Curtain Cap\"" w41 {
                        tunnel: w34 -> [w43 w53 w61 w71]
                        frame "Corona", Default {
                          n256 = local read "Curtain Cap Pol"() -> (w44:bool)
                          n257 = Number To Boolean Array(number=u16 0) -> (Boolean array=w50:bool[])
                          n258 = Replace Array Subset(array=w50, new element #1=w44, index #1=0 ("index"), new element #2=w43, index #2=1 ("index")) -> (w47:bool[])
                          n259 = Boolean Array To Number(Boolean array=w47) -> (number=w45:u16)
                          n260 = call "_Remote Communicate.vi"("DC Param"=w45, "Command"=_RT_Command."P1") -> ()  [unwired: 4 in, 4 out]
                        }
                        frame "Curtain Cap" {
                          n261 = local read "Corona Pol"() -> (w52:bool)
                          n262 = Number To Boolean Array(number=u16 0) -> (Boolean array=w59:bool[])
                          n263 = Replace Array Subset(array=w59, new element #1=w53, index #1=0 ("index"), new element #2=w52, index #2=1 ("index")) -> (w56:bool[])
                          n264 = Boolean Array To Number(Boolean array=w56) -> (number=w54:u16)
                          n265 = call "_Remote Communicate.vi"("DC Param"=w54, "Command"=_RT_Command."P1") -> ()  [unwired: 4 in, 4 out]
                        }
                        frame "Source 1" {
                          n266 = local read "Source 2 Pol"() -> (w62:bool)
                          n267 = Number To Boolean Array(number=u16 0) -> (Boolean array=w68:bool[])
                          n268 = Replace Array Subset(array=w68, new element #1=w61, index #1=0 ("index"), new element #2=w62, index #2=1 ("index")) -> (w65:bool[])
                          n269 = Boolean Array To Number(Boolean array=w65) -> (number=w63:u16)
                          n270 = call "_Remote Communicate.vi"("DC Param"=w63, "Command"=_RT_Command."P2") -> ()  [unwired: 4 in, 4 out]
                        }
                        frame "Source 2" {
                          n271 = local read "Source 1 Pol"() -> (w70:bool)
                          n272 = Number To Boolean Array(number=u16 0) -> (Boolean array=w77:bool[])
                          n273 = Replace Array Subset(array=w77, new element #1=w70, index #1=0 ("index"), new element #2=w71, index #2=1 ("index")) -> (w74:bool[])
                          n274 = Boolean Array To Number(Boolean array=w74) -> (number=w72:u16)
                          n275 = call "_Remote Communicate.vi"("DC Param"=w72, "Command"=_RT_Command."P2") -> ()  [unwired: 4 in, 4 out]
                        }
                      }
                      n276 = Format Into String(format string="Switch the %s channel to ", w41) -> (resulting string=w36:string)  [unwired: 2 in, 1 out]
                      n277 = Select(t="positive mode.", s=w34, f="negative mode.") -> (s? t:f=w37:string)
                      n278 = Concatenate Strings(w36, w37) -> (w35:string)
                      n279 = local write "String"(w35) -> ()
                      n280 = Not(x=w34) -> (.not. x?=w38:bool)
                    }
                    frame #2 {
                      n281 = case shown="\"Curtain Cap\"" w80 {
                        frame "Corona", Default {
                          n282 = local read "Corona +HV"() -> (w83:u16)
                          n283 = local read "Corona -HV"() -> (w84:u16)
                          n284 = call "_Remote Set PIC.vi"("Set Value"=w83, "PIC Channel"=_PIC_Channel."Corona +HV") -> ("error out"=w85:errorcluster)  [unwired: 1 in, 4 out]
                          n285 = call "_Remote Set PIC.vi"("error in (no error)"=w85, "Set Value"=w84, "PIC Channel"=_PIC_Channel."Corona -HV") -> ()  [unwired: 5 out]
                        }
                        frame "Curtain Cap" {
                          n286 = local read "Curtain Cap -HV"() -> (w89:u16)
                          n287 = local read "Curtain Cap +HV"() -> (w88:u16)
                          n288 = call "_Remote Set PIC.vi"("Set Value"=w88, "PIC Channel"=_PIC_Channel."Curtain Cap +HV") -> ("error out"=w90:errorcluster)  [unwired: 1 in, 4 out]
                          n289 = call "_Remote Set PIC.vi"("error in (no error)"=w90, "Set Value"=w89, "PIC Channel"=_PIC_Channel."Curtain Cap -HV") -> ()  [unwired: 5 out]
                        }
                        frame "Source 1" {
                          n290 = local read "Source 1 +HV"() -> (w94:u16)
                          n291 = local read "Source 1 -HV"() -> (w93:u16)
                          n292 = call "_Remote Set PIC.vi"("Set Value"=w94, "PIC Channel"=_PIC_Channel."Source 1 +HV") -> ("error out"=w95:errorcluster)  [unwired: 1 in, 4 out]
                          n293 = call "_Remote Set PIC.vi"("error in (no error)"=w95, "Set Value"=w93, "PIC Channel"=_PIC_Channel."Source 1 -HV") -> ()  [unwired: 5 out]
                        }
                        frame "Source 2" {
                          n294 = local read "Source 2 -HV"() -> (w99:u16)
                          n295 = local read "Source 2 +HV"() -> (w98:u16)
                          n296 = call "_Remote Set PIC.vi"("Set Value"=w98, "PIC Channel"=_PIC_Channel."Source 2 +HV") -> ("error out"=w100:errorcluster)  [unwired: 1 in, 4 out]
                          n297 = call "_Remote Set PIC.vi"("error in (no error)"=w100, "Set Value"=w99, "PIC Channel"=_PIC_Channel."Source 2 -HV") -> ()  [unwired: 5 out]
                        }
                      }
                      n298 = Format Into String(format string="Take the %s votage to a preset value and wait for %d mS.", w80, "Ramp Up T (mS)") -> (resulting string=w81:string)  [unwired: 2 in, 1 out]
                      n299 = local write "String"(w81) -> ()
                      n300 = Wait (ms)(milliseconds to wait="Ramp Up T (mS)") -> ()  [unwired: 1 out]
                    }
                  }
                  n301 = Increment(x=w17) -> (x+1=w13:i32)
                  "Current Cycle #" <- w13
                  n302 = Greater Or Equal?(x=w13, y="# of Cycles") -> (x >= y?=w15:bool)
                  n303 = Or(x="Abort Test", y=w15) -> (x .or. y?=w16:bool)
                }
              }
              frame #2 {
                w103 = FALSE
                n304 = property on="Abort Test" class="Bool (strict)"("Visible"=w103, "Value"=w103) -> ()  [unwired: 2 in, 2 out]
                n305 = property on="Start Test" class="Bool"("Visible"=TRUE) -> ()  [unwired: 2 in, 2 out]
              }
            }
          }
        }
        n306 = Wait (ms)(milliseconds to wait=u32 380) -> ()  [unwired: 1 out]
        n307 = local read "quit"() -> (w4:bool)
      }
    }
  }
